vi "WriteTree.vi"(8 "error in":errorcluster, 11 "repository in":refnum<class "NISE_CEF_HierarchyRepo.lvclass">) -> (0 "error out":errorcluster, 2 "root":T1, 3 "repository out":refnum<class "NISE_CEF_Repository.lvclass">)   [LabVIEW 2013, in "NISE_CEF_HierarchyRepo.lvclass"]
doc: "Transfers information between the repo and the tree control. This method should be called after the custom views are called or saving to disk."
uses:
  NISE_CEF_HierarchyRepo.lvclass
  Repository/NISE_CEF_Repository.lvclass
  Node/NodeRef.ctl
  Node/NISE_CEF_Node.lvclass
  Node/FromRepoCluster.ctl
  NISE_CEF_HierarchyRepo.lvclass/NISE_CEF_HierarchyRepo.ctl
  serializable node/NISE_CEF_serializable node.lvclass
  Node/NISE_CEF_Node.lvclass/NISE_CEF_Node.ctl
  Node/ReadChildren.vi
  tree serializer/NISE_CEF_TreeSerializer.lvlib
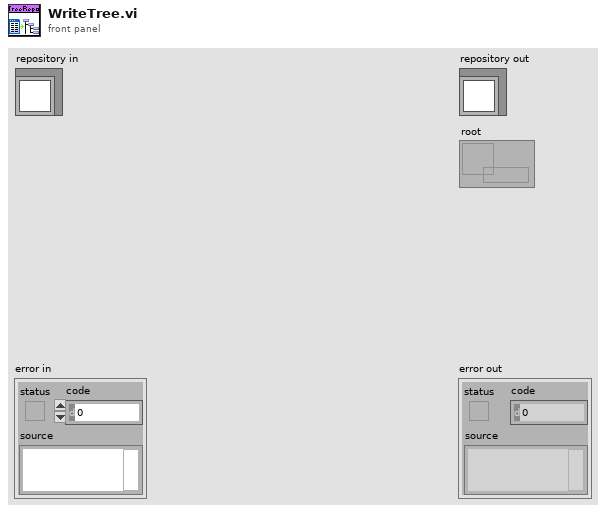
[diagram p1: front panel]
types:
  T1 = typedef "NISE_CEF_Node.lvclass/NodeRef.ctl" = refnum<data-value>
  T2 = typedef "NISE_CEF_Node.lvclass/FromRepoCluster.ctl" = cluster{"tag":string, "tags":string[], "classes":string[], "index":i32, "variant":variant}
  T3 = typedef "NISE_CEF_TreeSerializer.lvlib/memory hierarchy.ctl" = cluster{"hierarchy structure":T4, "instance data":refnum<class "NISE_CEF_serializable configuration.lvclass">[]}
  T4 = typedef "NISE_CEF_TreeSerializer.lvlib/full hierarchy.ctl" = cluster{"root":string, "hierarchy":T5[]}
  T5 = typedef "NISE_CEF_TreeSerializer.lvlib/hierarchy element.ctl" = cluster{"current node":string, "children":string[]}
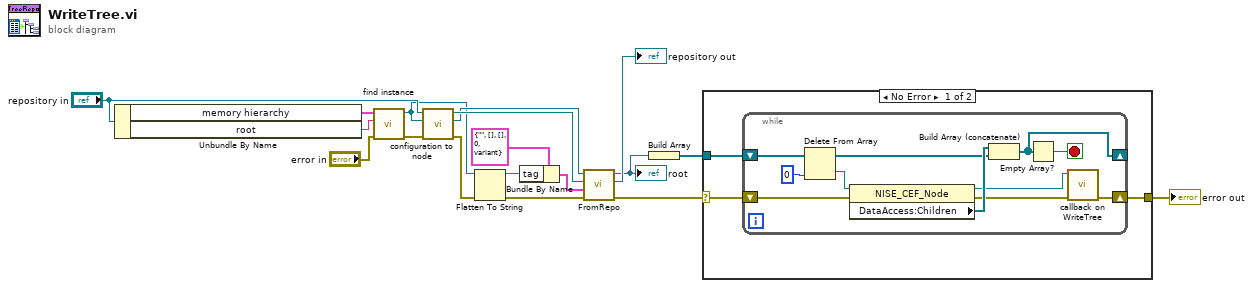
[diagram p0: block diagram]
diagram:
  n1 = Unbundle By Name("repository in") -> ("memory hierarchy"=w15:T3, "root"=w17:string)
  n2 = call "find instance.vi"("error in"="error in", "ID"=w17, "memory hierarchy"=w15) -> ("error out"=w10:errorcluster, "configuration"=w6:refnum<class "NISE_CEF_serializable configuration.lvclass">)  [unwired: 7 in]
  n3 = call-dynamic "configuration to node.vi"("error in"=w10, "configuration"=w6, "hierarchy repo in"="repository in") -> ("error out"=w11:errorcluster, "node"=w12:refnum<class "NISE_CEF_serializable node.lvclass">, "hierarchy repo out"=w13:refnum<class "NISE_CEF_HierarchyRepo.lvclass">)  [unwired: 6 in]
  n4 = Flatten To String(anything=w6, error in (no error)=w11) -> (data string=w5:string, error out=w7:errorcluster)  [unwired: 2 in, 1 out]
  n5 = Bundle By Name(cluster=T2 {"tag"="", "tags"=[], "classes"=[], "index"=0, "variant"=variant} ("from repo cluster"), "tag"=w5) -> (w8:T2)
  n6 = call-dynamic "FromRepo.vi"("error in"=w7, "from repo cluster"=w8, "repository in"=w13, "node in"=w12) -> ("error out"=w4:errorcluster, "repository out"=→"repository out":refnum<class "NISE_CEF_Repository.lvclass">, "node"=w2:T1)  [unwired: 5 in]
  "root" <- w2
  n7 = Build Array(w2) -> (w1:T1[])
  n8 = case shown="No Error" w4 {
    selector: w4 -> [w21 w33]
    tunnel: [w20 w33] -> w3
    tunnel: w1 -> [w19 _]
    frame No Error {
      n9 = while {
        shift-right: [w22] -> w20
        shift-left: w21 -> [w30]
        shift-right: [w26] -> _
        shift-left: w19 -> [w32]
        stop <- w25 stop-if-true
        n10 = Delete From Array(array=w32, index=0) -> (deleted portion=w29:T1, array with subset deleted=w27:T1[])  [unwired: 1 in]
        n11 = property class="NISE_CEF_Node"(reference=w29, error in=w30) -> (reference out=w24:T1, error out=w23:errorcluster, "DataAccess:Children"=w28:T1[])
        n12 = Build Array (concatenate)(w28, w27) -> (w26:T1[])
        n13 = Empty Array?(array=w26) -> (empty?=w25:bool)
        n14 = call "callback on WriteTree.vi"("error in"=w23, "node"=w24) -> ("error out"=w22:errorcluster)  [unwired: 9 in]
      }
    }
    frame Error {
    }
  }
  "error out" <- w3
